vi "Generate LV Icon Template Layer.vi"(6 "Text settings":T1={"Font"="Small Fonts", "Alignment"=1, "Size"=8, "Center text"=TRUE, "Capitalize text"=TRUE, "Text color"={"Line 1 color"=0, "Line 2 color"=0, "Line 3 color"=0, "Line 4 color"=0}} {"Alignment" items=["left", "center", "right"]}, 7 "Text":T4, 8 "error in (no error)":errorcluster, 10 "Template path":path, 11 "Icon.lvclass in":refnum<class "Icon.lvclass">) -> (0 "error out":errorcluster, 3 "Icon.lvclass out":refnum<class "Icon.lvclass">)   [LabVIEW 2020, in "LabVIEW Icon API.lvlib"]
doc: "Generating the LV Icon Template Layer requires the Template path to the glyph. This path has to be a fully qualified path.\nIn addition to the path, it is possible to specify the Text as well as the visual appearance of the text.\n\nThe default value of Text is an empty string for all four lines.\nThe default value for the visual appearance is:\nFont: Small Fonts\nAlignment: Center\nSize: 8\nCenter text vertically: TRUE\nCapitalize text: TRUE\nColor of all four lines: Black"
uses:
  <vilib>/LabVIEW Icon API/LabVIEW Icon API.lvlib
  <vilib>/LabVIEW Icon API/lv_icon/Classes/Icon/Icon.lvclass
  <vilib>/LabVIEW Icon API/API_Text.ctl
  <vilib>/LabVIEW Icon API/API_Test Settings.ctl
  <vilib>/LabVIEW Icon API/lv_icon/Controls/Alignment.ctl
  <vilib>/LabVIEW Icon API/API_Text Colors.ctl
  <vilib>/LabVIEW Icon API/lv_icon/Controls/Graphic.ctl
  <vilib>/LabVIEW Icon API/lv_icon/Classes/Icon Framework/Icon Framework.lvclass
  <vilib>/LabVIEW Icon API/lv_icon/lv_icon.lvlib
panel:
  in  "Template Layer":string="Template"
  in  "LayerName":string="Icon Text"
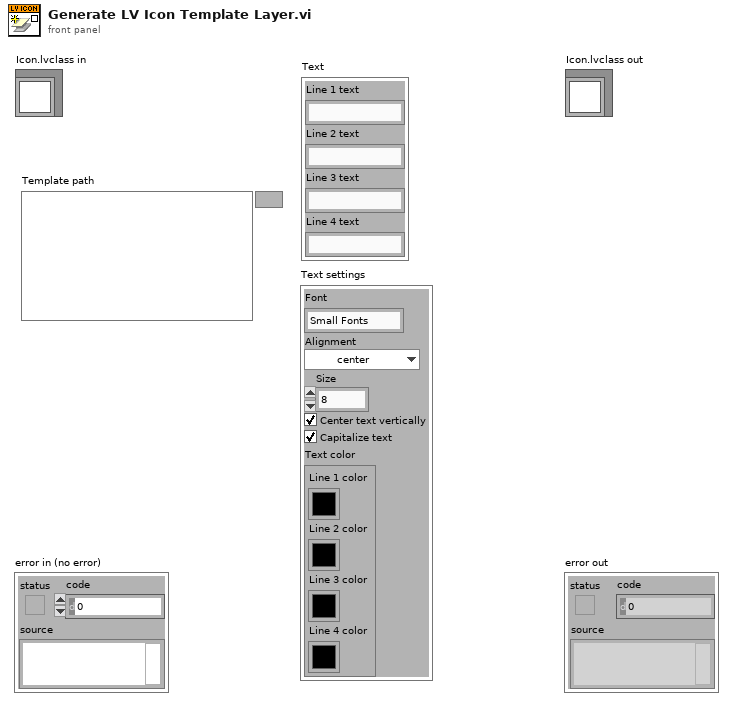
[diagram p1: front panel]
types:
  T1 = typedef "LabVIEW Icon API.lvlib/API_Test Settings.ctl" = cluster{"Font":string, "Alignment":T2, "Size":u8, "Center text":bool, "Capitalize text":bool, "Text color":T3}
  T2 = typedef "Alignment.ctl" = u16
  T3 = typedef "LabVIEW Icon API.lvlib/API_Text Colors.ctl" = cluster{"Line 1 color":u32, "Line 2 color":u32, "Line 3 color":u32, "Line 4 color":u32}
  T4 = typedef "LabVIEW Icon API.lvlib/API_Text.ctl" = cluster{"Line 1 text":string, "Line 2 text":string, "Line 3 text":string, "Line 4 text":string}
  T5 = typedef "Graphic.ctl" = cluster{"Rectangle":cluster{"left":i16, "top":i16, "right":i16, "bottom":i16}, "Path":path, "Image":picture, "Filter":string, "FileName":string}
  T6 = typedef "BodyText.ctl" = cluster{"Line 1 text":string, "Line 2 text":string, "Line 3 text":string, "Line 4 text":string, "Line 1 color":u32, "Line 2 color":u32, "Line 3 color":u32, "Line 4 color":u32, "Body Text Spec":cluster{"Font":T7, "Alignment":T2, "Size":u8}, "Center text vertically":bool, "Capitalize Text":bool}
  T7 = typedef "Font.ctl" = string
  T8 = typedef "imagedata.ctl" = cluster{"image type":i32, "image depth":i32, "image":u8[], "mask":u8[], "colors":u32[], "Rectangle":cluster{"left":i16, "top":i16, "right":i16, "bottom":i16}}
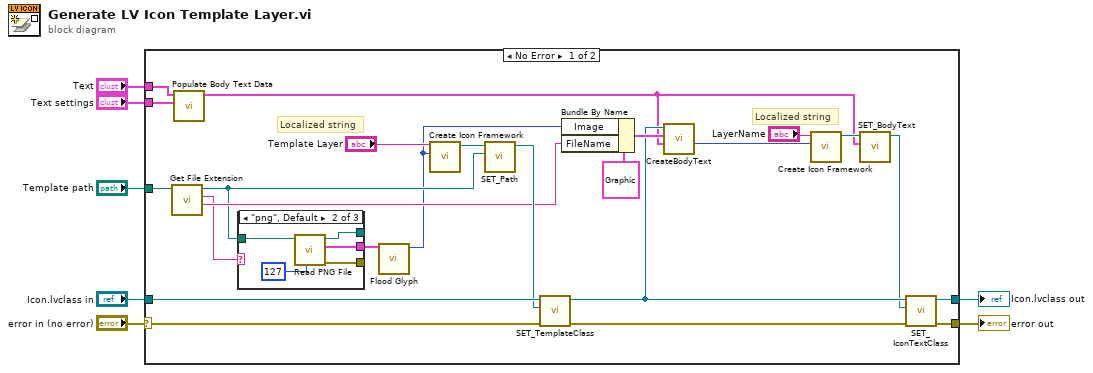
[diagram p0: block diagram]
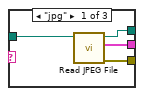
[diagram p2: hidden frame]
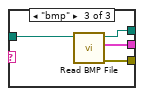
[diagram p3: hidden frame]
diagram:
  n1 = case shown="No Error" "error in (no error)" {
    selector: "error in (no error)" -> [w24 w46]
    tunnel: [w19 w46] -> w6
    tunnel: "Icon.lvclass in" -> [w22 w45]
    tunnel: "Text settings" -> [w31 _]
    tunnel: "Text" -> [w30 _]
    tunnel: [w18 w45] -> w2
    tunnel: "Template path" -> [w16 _]
    frame No Error {
      # "Localized string"
      # "Localized string"
      n2 = call <vilib>:"Get File Extension.vi"("file"=w16) -> ("filename without extension"=w15:string, "lowercase file extension"=w13:string, "dup file"=w12:path)  [unwired: 6 in, 2 out]
      n3 = call <vilib>:"Populate Body Text Data.vi"("Text settings"=w31, "Text"=w30) -> ("Body Text"=w8:T6)  [unwired: 9 in]
      n4 = case shown="\"png\", Default" w13 {
        tunnel: [w35 w40 w44] -> _
        tunnel: [w34 w39 w43] -> w14
        tunnel: [w33 w38 w42] -> _
        tunnel: w12 -> [w32 w36 w41]
        frame "jpg" {
          n5 = call <vilib>:"Read JPEG File.vi"("path to JPEG file"=w32) -> ("error out"=w35:errorcluster, "image data"=w34:T8, "path"=w33:path)  [unwired: 1 in, 7 out]
        }
        frame "png", Default {
          n6 = call <vilib>:"Read PNG File.vi"("Transparency Thresh"=u8 127, "path to PNG file"=w36) -> ("error out"=w40:errorcluster, "image data"=w39:T8, "path"=w38:path)  [unwired: 1 in, 6 out]
        }
        frame "bmp" {
          n7 = call <vilib>:"Read BMP File.vi"("path to BMP file"=w41) -> ("error out"=w44:errorcluster, "image data"=w43:T8, "path"=w42:path)  [unwired: 1 in, 7 out]
        }
      }
      n8 = call <vilib>:"Flood Glyph.vi"("image data"=w14) -> ("Pic Out"=w11:picture)  [unwired: 1 in, 9 out]
      n9 = call <vilib>:"Create Icon Framework.vi"("Template Glyph"=w11, "Layer name"="Template Layer") -> ("Icon Framework out"=w23:refnum<class "Icon Framework.lvclass">)  [unwired: 9 in]
      n10 = call <vilib>:"SET_Path.vi"("Path"=w12, "Icon Framework.lvclass in"=w23) -> ("Icon Framework.lvclass out"=w21:refnum<class "Icon Framework.lvclass">)  [unwired: 8 in, 1 out]
      n11 = call-dynamic "SET_TemplateClass.vi"("error in (no error)"=w24, "Icon Framework.lvclass"=w21, "Icon.lvclass in"=w22) -> ("error out"=w20:errorcluster, "Icon.lvclass out"=w17:refnum<class "Icon.lvclass">)  [unwired: 7 in]
      n12 = Bundle By Name(cluster=T5 {"Rectangle"={"left"=0, "top"=0, "right"=0, "bottom"=0}, "Path"=path "", "Image"=bytes[0], "Filter"="", "FileName"=""} ("Path and Icon Template"), "Image"=w11, "FileName"=w15) -> (w28:T5)
      n13 = call <vilib>:"CreateBodyText.vi"("Body Text"=w8, "Path and Icon Template"=w28, "Icon.lvclass in"=w17) -> ("Body Text"=w26:picture)  [unwired: 8 in]
      n14 = call <vilib>:"Create Icon Framework.vi"("Template Glyph"=w26, "Layer name"="LayerName") -> ("Icon Framework out"=w10:refnum<class "Icon Framework.lvclass">)  [unwired: 9 in]
      n15 = call-dynamic "SET_BodyText.vi"("Body Text"=w8, "Icon Framework.lvclass in"=w10) -> ("Icon Framework.lvclass out"=w9:refnum<class "Icon Framework.lvclass">)  [unwired: 8 in, 1 out]
      n16 = call-dynamic "SET_IconTextClass.vi"("error in (no error)"=w20, "Icon Framework.lvclass"=w9, "Icon.lvclass in"=w17) -> ("error out"=w19:errorcluster, "Icon.lvclass out"=w18:refnum<class "Icon.lvclass">)  [unwired: 7 in]
    }
    frame Error {
    }
  }
  "error out" <- w6
  "Icon.lvclass out" <- w2
